vi "TL simulate the boat.vi"(1 "Boat Speed\npixels/sec":dbl=2.0 format="%#_13g", 2 "Rudder":dbl, 3 "Loop time":u32=200, 4 "GPS":cluster{"X pos":i32, "Y pos":i32, "Heading":dbl}={"X pos"=200, "Y pos"=250, "Heading"=0.0}) -> (0 "GPS out":cluster{"X pos":i32, "Y pos":i32, "Heading":dbl})   [LabVIEW 2014]
panel:
  out "motion\npixels":dbl
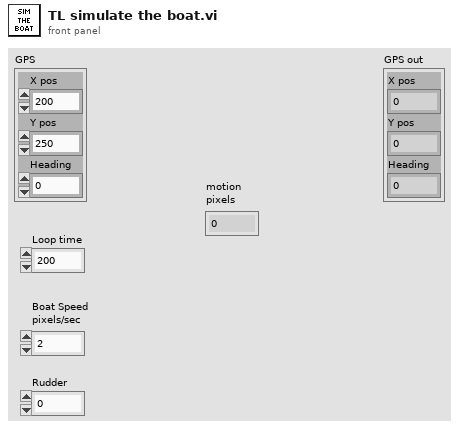
[diagram p1: front panel]
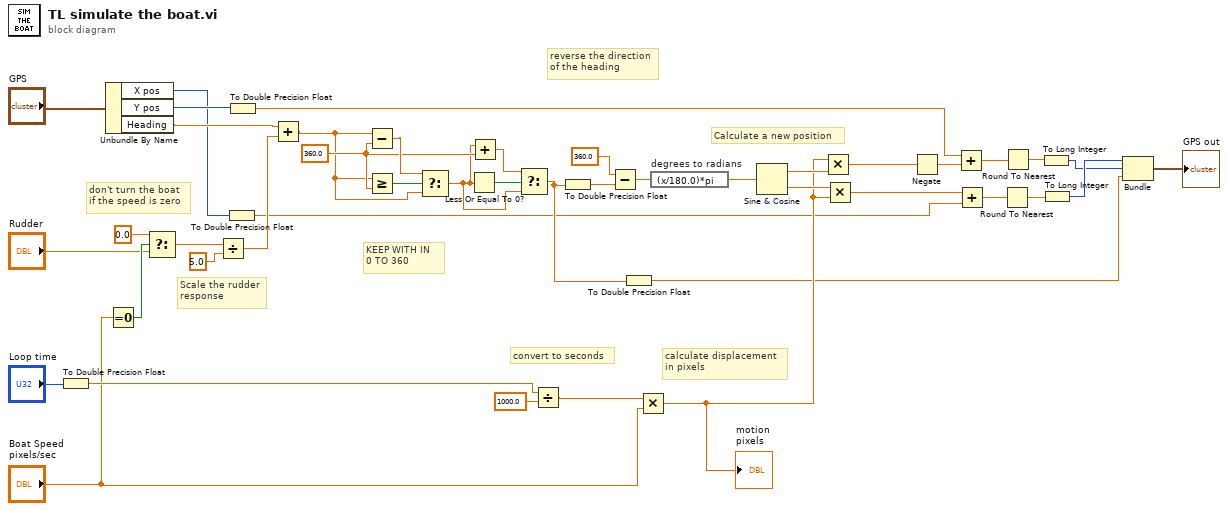
[diagram p0: block diagram]
diagram:
  w34 = 360.0
  # "Scale the rudder\nresponse"
  # "don't turn the boat\nif the speed is zero"
  # "reverse the direction\nof the heading"
  # "KEEP WITH IN \n0 TO 360"
  # "Calculate a new position"
  # "calculate displacement\nin pixels"
  # "convert to seconds"
  n1 = To Double Precision Float(number="Loop time") -> (double precision float=w28:dbl)
  n2 = Unbundle By Name("GPS") -> ("X pos"=w16:i32, "Y pos"=w18:i32, "Heading"=w20:dbl)
  n3 = Equal To 0?(x="Boat Speed\npixels/sec") -> (x = 0?=w10:bool)
  n4 = Select(t=0.0, s=w10, f="Rudder") -> (s? t:f=w7:dbl)
  n5 = Divide(x=w7, y=5.0) -> (x/y=w19:dbl)
  n6 = To Double Precision Float(number=w16) -> (double precision float=w15:dbl)
  n7 = To Double Precision Float(number=w18) -> (double precision float=w17:dbl)
  n8 = Add(x=w20, y=w19) -> (x+y=w31:dbl)
  n9 = Subtract(x=w31, y=w34) -> (x-y=w36:dbl)
  n10 = Greater Or Equal?(x=w31, y=w34) -> (x >= y?=w37:bool)
  n11 = Select(t=w36, s=w37, f=w31) -> (s? t:f=w32:dbl)
  n12 = Less Or Equal To 0?(x=w32) -> (x <= 0?=w35:bool)
  n13 = Add(x=w32, y=w34) -> (x+y=w33:dbl)
  n14 = Select(t=w33, s=w35, f=w32) -> (s? t:f=w22:dbl)
  n15 = Divide(x=w28, y=1000.0) -> (x/y=w27:dbl)
  n16 = To Double Precision Float(number=w22) -> (double precision float=w38:dbl)
  n17 = Subtract(x=360.0, y=w38) -> (x-y=w40:dbl)
  n18 = To Double Precision Float(number=w22) -> (double precision float=w21:dbl)
  n19 = Multiply(x=w27, y="Boat Speed\npixels/sec") -> (x*y=w24:dbl)
  "motion\npixels" <- w24
  n20 = expression code="(x/180.0)*pi" "degrees to radians"(w40) -> (w43:dbl)
  n21 = Sine & Cosine(0:w43) -> (1:w42:dbl, 2:w41:dbl)
  n22 = Multiply(x=w24, y=w42) -> (x*y=w13:dbl)
  n23 = Multiply(x=w41, y=w24) -> (x*y=w14:dbl)
  n24 = Negate(x=w13) -> (-x=w26:dbl)
  n25 = Add(x=w17, y=w26) -> (x+y=w4:dbl)
  n26 = Add(x=w14, y=w15) -> (x+y=w6:dbl)
  n27 = Round To Nearest(number=w6) -> (nearest integer value=w5:dbl)
  n28 = Round To Nearest(number=w4) -> (nearest integer value=w3:dbl)
  n29 = To Long Integer(number=w3) -> (32bit integer=w11:i32)
  n30 = To Long Integer(number=w5) -> (32bit integer=w12:i32)
  n31 = Bundle(w12, w11, w21) -> (→"GPS out":cluster{i32, i32, dbl})  [unwired: 1 in]
